vi "Update UI.vi"(8 "error in (no error)":errorcluster, 10 "string":string, 11 "Connection Listener in":refnum<class "Connection Listener.lvclass">) -> (0 "error out":errorcluster, 3 "Connection Listener out":refnum<class "Connection Listener.lvclass">)   [LabVIEW 2017, in "Connection Listener.lvlib" / "Connection Listener.lvclass"]
uses:
  Connection Listener.lvclass
  Connection Listener.lvclass/Connection Listener.ctl
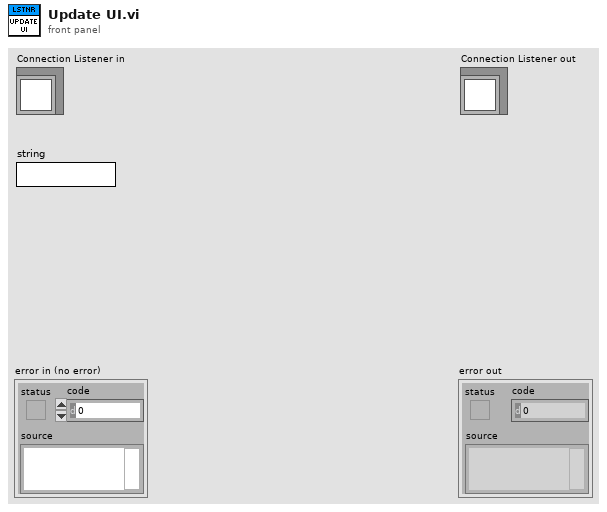
[diagram p1: front panel]
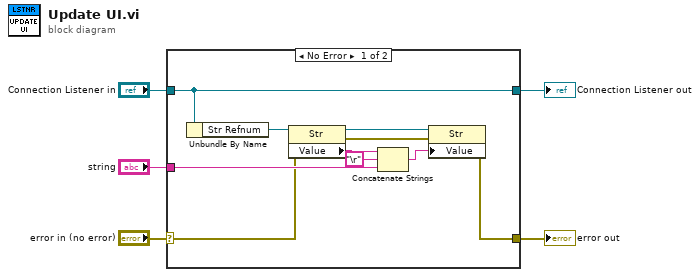
[diagram p0: block diagram]
diagram:
  n1 = case shown="No Error" "error in (no error)" {
    selector: "error in (no error)" -> [w7 w17]
    tunnel: [w6 w17] -> w4
    tunnel: [w15 w16] -> w2
    tunnel: "Connection Listener in" -> [w15 w16]
    tunnel: "string" -> [w10 _]
    frame No Error {
      n2 = Unbundle By Name(w15) -> ("Str Refnum"=w14:refnum<vi>)
      n3 = property class="Str"(reference=w14, error in=w7) -> (reference out=w13:refnum<vi>, error out=w8:errorcluster, "Value"=w12:string)
      n4 = Concatenate Strings(w12, "\r", w10) -> (w11:string)
      n5 = property class="Str"(reference=w13, error in=w8, "Value"=w11) -> (error out=w6:errorcluster)  [unwired: 1 out]
    }
    frame Error {
    }
  }
  "error out" <- w4
  "Connection Listener out" <- w2
